vi "spin_to_color.vi"(7 "Description":string, 8 "Command Info In":T1, 10 "Color":enum16{"red", "blue", "yellow", "green"}(ring)) -> (0 "Command Info Out":T1)   [LabVIEW 2019]
doc: "This template is useful for immediate subsystem actions that do not need deadband filtering\n\nBe sure to right-click and select New from Template and save with a new command name."
uses:
  <vilib>/Rock Robotics/WPI/Framework/Command Status Info.ctl
  <vilib>/Rock Robotics/WPI/Framework/Completion Status.ctl
  <vilib>/Rock Robotics/WPI/Framework/Completion Notifier.ctl
  Implementation/ColorSensor Setpoints.ctl
  Implementation/ColorSensor Operations.ctl
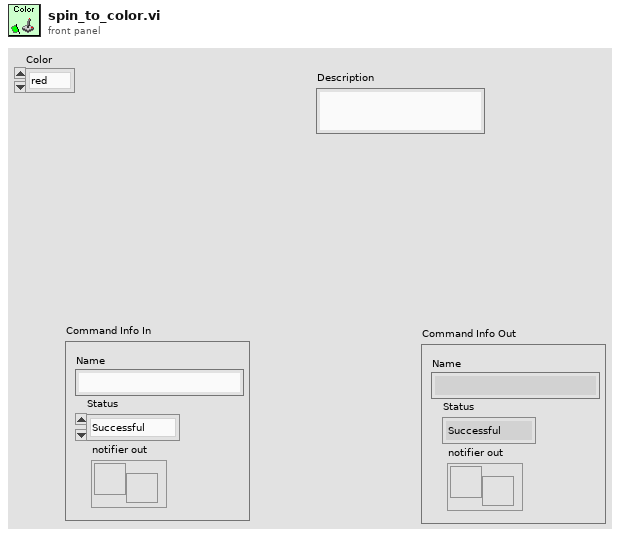
[diagram p1: front panel]
types:
  T1 = typedef "Command Status Info.ctl" = cluster{"Name":string, "Status":T2, "notifier out":T3}
  T2 = typedef "Completion Status.ctl" = enum16{"Successful", "Aborted", "Incomplete"}
  T3 = typedef "Completion Notifier.ctl" = refnum<notifier>
  T4 = typedef "ColorSensor Setpoints.ctl" = cluster{"Operation":T5, "Rotations":dbl, "Color":enum16{"red", "blue", "yellow", "green"}}
  T5 = typedef "ColorSensor Operations.ctl" = enum16{"Reserve", "Read Current", "spin_to_color", "ColorSpin", "Immediate", "Stop"}
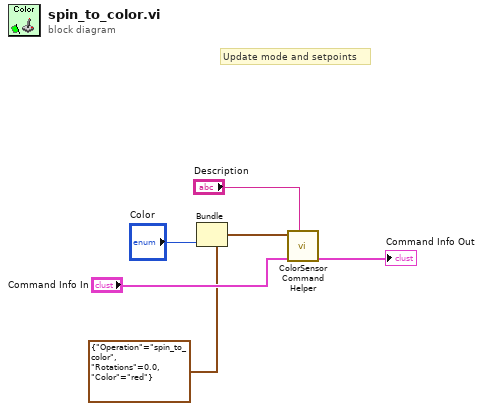
[diagram p0: block diagram]
diagram:
  # "Update mode and setpoints"
  n1 = Bundle(cluster=T4 {"Operation"=enum."spin_to_color", "Rotations"=0.0, "Color"=enum."red"} ("Default Command"), "Color"="Color") -> (w3:T4)  [unwired: 2 in]
  n2 = call "ColorSensor Command Helper.vi"("Description"="Description", "Command Info In"="Command Info In", "SubSystem Data"=w3) -> ("Command Info Out"=→"Command Info Out":T1)  [unwired: 6 in, 2 out]
